vi "HTTP Server.vi"(11 "HTTPServerService in":refnum<class "HTTPServerService.lvclass">) -> (2 "HTTP Server":refnum<class "Server.lvclass">)   [LabVIEW 2020, in "Vecto.lvlib" / "HTTPServerService.lvclass"]
uses:
  HTTPServerService.lvclass
  <vilib>/IlluminatedG/IG HTTP Server/HTTP Server/Server/Server.lvclass
  HTTPServerService.lvclass/HTTPServerService.ctl
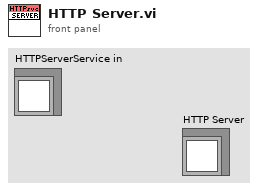
[diagram p1: front panel]
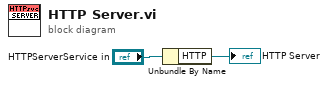
[diagram p0: block diagram]
diagram:
  n1 = Unbundle By Name("HTTPServerService in") -> ("HTTP"=→"HTTP Server":refnum<class "Server.lvclass">)
